vi "Redirect to Subscriber.vi"(8 "error in (no error)":errorcluster, 10 "WebSocket Service Data Handler Msg":refnum<class "WebSocket Service Connection Handler Msg.lvclass">, 11 "WebSocket Service Actor in":refnum<class "WebSocket Service.lvclass">) -> (0 "error out":errorcluster, 3 "WebSocket Service Actor out":refnum<class "WebSocket Service.lvclass">)   [LabVIEW 2016, in "WebSocket Actors.lvlib" / "WebSocket Service.lvclass"]
uses:
  WebSocket Service.lvclass
  WebSocket Service Messages/WebSocket Service Connection Handler Msg/WebSocket Service Connection Handler Msg.lvclass
  C:/Projects/Shared Libraries/WebSocket Actor/WebSocket Actor/Abstract Messages/WebSocket Connection Handler Msg/WebSocket Connection Handler Msg.lvclass
  WebSocket Service.lvclass/WebSocket Service.ctl
  Abstract Messages/WebSocket Connection Handler Msg/WebSocket Connection Handler Msg.lvclass/WebSocket Connection Handler Msg.ctl
  <vilib>/ActorFramework/Message Enqueuer/Message Enqueuer.lvclass/Message Enqueuer.ctl
  Abstract Messages/WebSocket Connection Handler Msg/properties/Read Connection Event.vi
  Abstract Messages/WebSocket Connection Handler Msg/properties/Read Peer ID.vi
  Abstract Messages/WebSocket Connection Handler Msg/properties/Read Data.vi
  <vilib>/ActorFramework/Message Enqueuer/Enqueue.vi
  Abstract Messages/WebSocket Connection Handler Msg/WebSocket Connection Handler Msg.lvclass
  C:/Program Files (x86)/National Instruments/LabVIEW 2016/vi.lib/ActorFramework/Message/Message.lvclass
  <vilib>/ActorFramework/Message Priority Queue/Priority Enqueue.vi
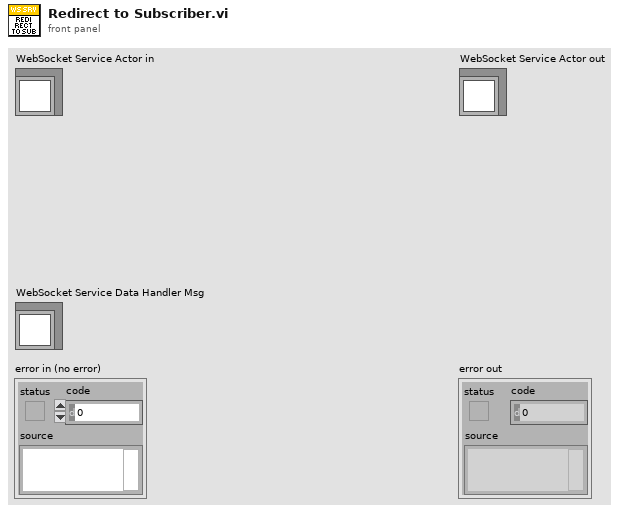
[diagram p1: front panel]
types:
  T1 = typedef "WebSocket Actors.lvlib/WebSocket Connection Handler Msg.lvclass/Connection Event.ctl" = enum16{"On Connect", "On Message", "On Close"}
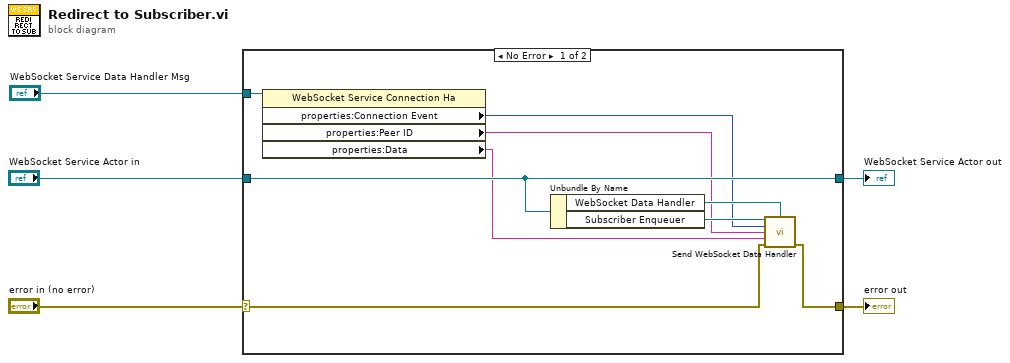
[diagram p0: block diagram]
diagram:
  n1 = case shown="No Error" "error in (no error)" {
    selector: "error in (no error)" -> [w11 w16]
    tunnel: [w10 w16] -> w4
    tunnel: [w14 w15] -> w2
    tunnel: "WebSocket Service Actor in" -> [w14 w15]
    tunnel: "WebSocket Service Data Handler Msg" -> [w9 _]
    frame No Error {
      n2 = property class="WebSocket Service Connection Ha"(reference=w9) -> ("properties:Connection Event"=w8:T1, "properties:Peer ID"=w7:string, "properties:Data"=w6:string)  [unwired: 1 in, 2 out]
      n3 = Unbundle By Name(w14) -> ("WebSocket Data Handler"=w12:refnum<class "WebSocket Connection Handler Msg.lvclass">, "Subscriber Enqueuer"=w13:refnum<class "Message Enqueuer.lvclass">)
      n4 = call "Send WebSocket Data Handler.vi"("Message Enqueuer"=w13, "Message Type"=w12, "Connection Event"=w8, "Peer ID"=w7, "Data"=w6, "error in (no error)"=w11) -> ("error out"=w10:errorcluster)  [unwired: 8 in, 1 out]
    }
    frame Error {
    }
  }
  "error out" <- w4
  "WebSocket Service Actor out" <- w2
